vi "PQregisterThreadLock.vi"(8 "error in (no error)":errorcluster) -> (0 "error out":errorcluster, 3 "return type":u32)   [LabVIEW 2019, in "libpqlv.lvlib"]
uses:
  libpqlv.lvlib
  libpq.dll
panel:
  in  "newhandler":u32
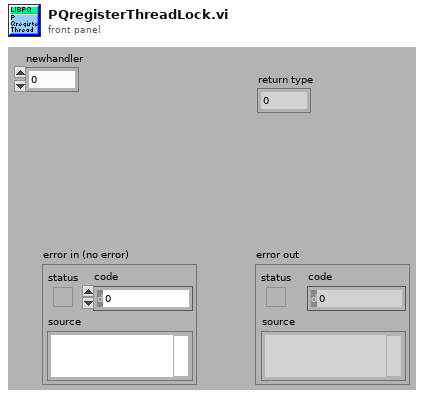
[diagram p1: front panel]
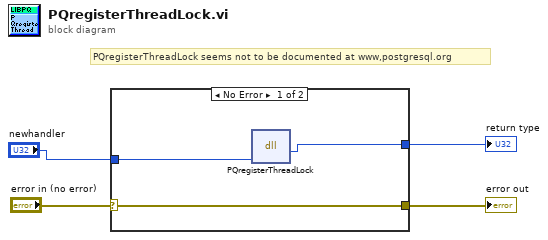
[diagram p0: block diagram]
diagram:
  # "PQregisterThreadLock seems not to be documented at www,postgresql.org"
  n1 = case shown="No Error" "error in (no error)" {
    selector: "error in (no error)" -> [w7 w8]
    tunnel: [w7 w8] -> w3
    tunnel: [w6 _] -> w2
    tunnel: "newhandler" -> [w5 _]
    frame No Error {
      n2 = dll-call lib="libpq.*" fn="PQregisterThreadLock"("newhandler"=w5) -> ("PQregisterThreadLock"=w6:u32)  [unwired: 4 in, 2 out]
    }
    frame Error {
    }
  }
  "return type" <- w2
  "error out" <- w3
